vi "D-Type Flip-Flop.vi"(2 "clock":bool, 3 "Data":bool=TRUE) -> (0 "!Q":bool, 1 "Q":bool=TRUE)   [LabVIEW 2018]
panel:
  # "D-Type Flip-Flop.\n\nThis can be used as a Functional Global Variable or\nto run it now;\n-Click run continuously\n-Choose whether to have data high or low with the \n  data button.\n-Click the clock button to clock the data through.\n-To stop the VI click the run continuously button\n again."
  # "D-Type\nFlip-Flop"
  # "Truth Table\n\nClock \t        D    \tQ     Qprev\nRising edge \t0    \t0 \t       X\nRising edge \t1 \t   1 \t       X\nNon-Rising \t X  \tQprev"
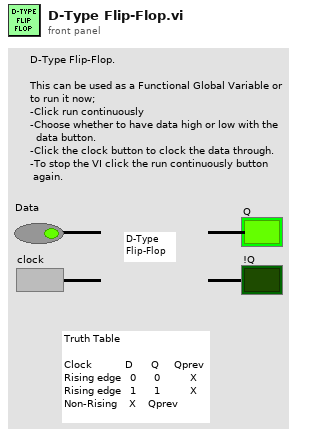
[diagram p1: front panel]
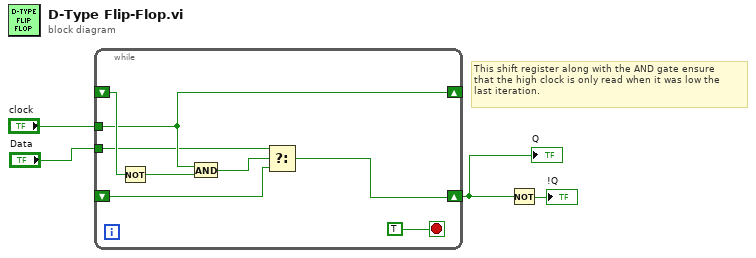
[diagram p0: block diagram]
diagram:
  # "This shift register along with the AND gate ensure\nthat the high clock is only read when it was low the \nlast iteration."
  n1 = while {
    shift-right: [w6] -> _
    shift-left: _ -> [w11]
    shift-right: [w8] -> w3
    shift-left: _ -> [w7]
    tunnel: "clock" -> [w6]
    tunnel: "Data" -> [w5]
    stop <- TRUE stop-if-true
    n2 = Not(x=w11) -> (.not. x?=w10:bool)
    n3 = And(x=w6, y=w10) -> (x .and. y?=w9:bool)
    n4 = Select(t=w5, s=w9, f=w7) -> (s? t:f=w8:bool)
  }
  "Q" <- w3
  n5 = Not(x=w3) -> (.not. x?=→"!Q":bool)
